vi "adad.vi"(7 "error in":errorcluster) -> (27 "error out":errorcluster)   [LabVIEW 2021]
uses:
  <vilib>/vision/NI_Vision_Development_Module.lvlib
panel:
  out "Image Out":T1(plugin-control)
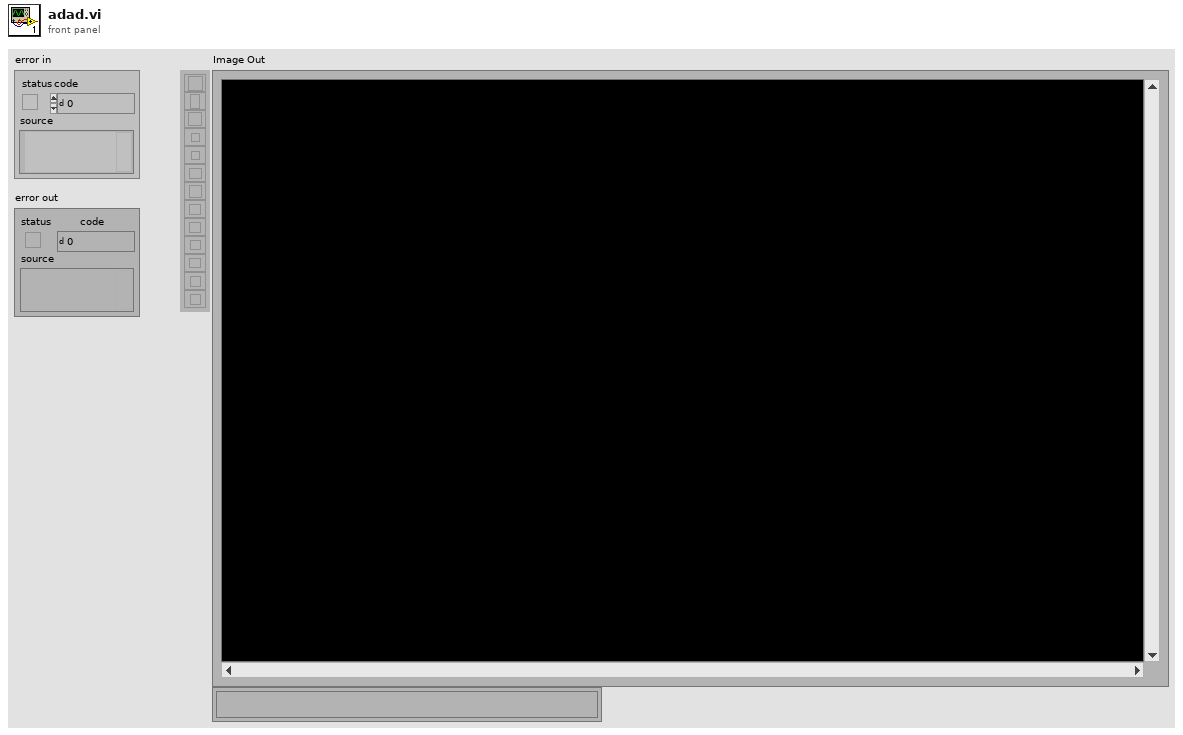
[diagram p1: front panel]
types:
  T1 = typedef "IMAQ Image.ctl" = refnum<image>
  T2 = typedef "Image Type" = u32
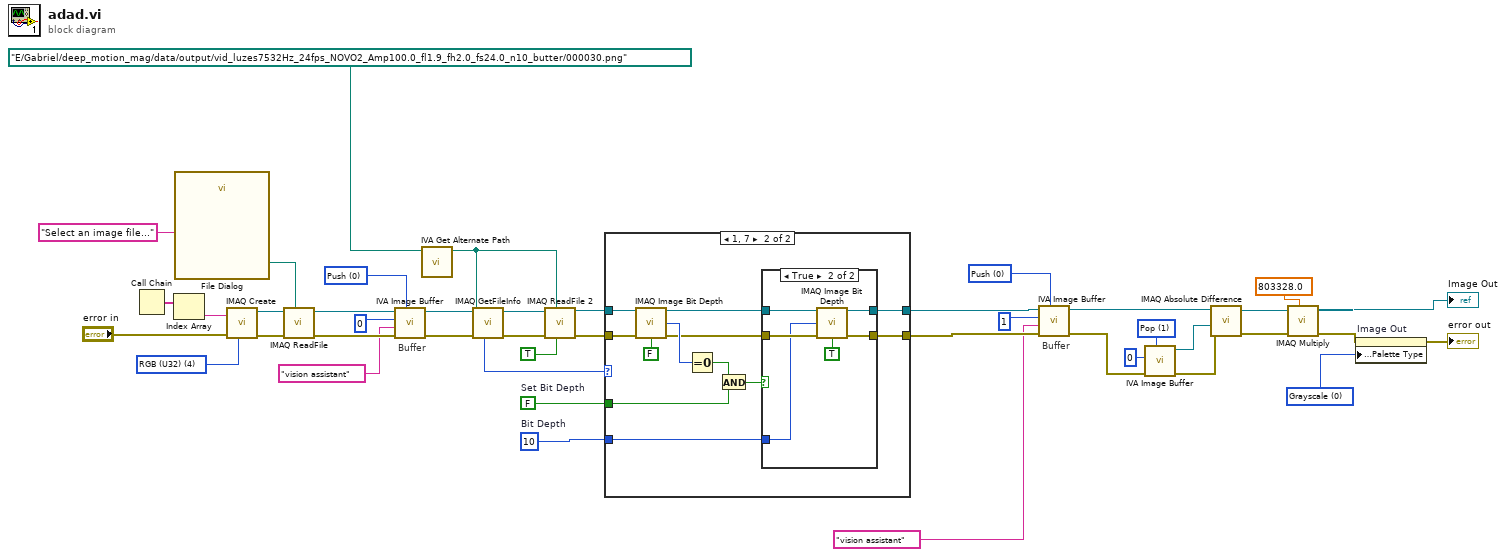
[diagram p0: block diagram]
diagram:
  w1 = u32 0 items=["Grayscale", "Binary", "Gradient", "Rainbow", "Temperature", "User Defined", "Binary 16 Bit", "Gradient 16 Bit", "Rainbow 16 Bit", "Temperature 16 Bit", "User Defined 16 Bit"] ("Palette Type")
  w12 = u16 1 items=["Push", "Pop", "Reset"] ("Function")
  w15 = u16 0 items=["Push", "Pop", "Reset"] ("Function")
  w25 = 10  # Bit Depth
  w26 = FALSE  # Set Bit Depth
  w31 = u16 0 items=["Push", "Pop", "Reset"] ("Function")
  w34 = T2 4 items=["Grayscale (U8)", "Grayscale (I16)", "Grayscale (SGL)", "Complex (CSG)", "RGB (U32)", "HSL (U32)", "RGB (U64)", "Grayscale (U16)"] ("Image Type")
  # "Buffer"
  # "Buffer"
  n1 = Call Chain() -> (call chain=w38:string[])
  n2 = Index Array(array=w38) -> (element=w37:string)  [unwired: 1 in]
  n3 = call "File Dialog"("prompt"="Select an image file...") -> ("selected path"=w35:path)  [unwired: 6 in, 8 out]
  n4 = call "IMAQ Create"("Image Name"=w37, "Image Type"=w34, "error in (no error)"="error in") -> ("New Image"=w41:T1, "error out"=w40:errorcluster)  [unwired: 1 in, 1 out]
  n5 = call "IMAQ ReadFile"("File Path"=w35, "error in (no error)"=w40, "Image"=w41) -> ("error out"=w42:errorcluster, "Image Out"=w33:T1)  [unwired: 2 in, 5 out]
  n6 = call <vilib>:"IVA Image Buffer.vi"("Function"=w31, "error in (no error)"=w42, "Prefix"="vision assistant", "Buffer #"=0, "Image In"=w33) -> ("error out"=w32:errorcluster, "Image Out"=w23:T1)  [unwired: 5 out]
  n7 = call <vilib>:"IVA Get Alternate Path.vi"("Path In"=path "E:/Gabriel/deep_motion_mag/data/output/vid_luzes7532Hz_24fps_NOVO2_Amp100.0_fl1.9_fh2.0_fs24.0_n10_butter/000030.png" ("File Path")) -> ("Path Out"=w21:path)  [unwired: 10 out]
  n8 = call "IMAQ GetFileInfo"("error in (no error)"=w32, "File Path"=w21) -> ("error out"=w19:errorcluster, "Image Type"=w27:T2)  [unwired: 8 out]
  n9 = call "IMAQ ReadFile 2"("Use File Path Image Type"=TRUE, "File Path"=w21, "error in (no error)"=w19, "Image"=w23) -> ("error out"=w20:errorcluster, "Image Out"=w22:T1)  [unwired: 3 in, 3 out]
  n10 = case shown="1, 7" w27 {
    tunnel: w22 -> [w44 w53]
    tunnel: w20 -> [w43 w52]
    tunnel: w26 -> [_ w46]
    tunnel: w25 -> [_ w56]
    tunnel: [w44 w55] -> w17
    tunnel: [w43 w54] -> w24
    frame 0, Default {
    }
    frame 1, 7 {
      n11 = call "IMAQ Image Bit Depth"("Image"=w53, "error in (no error)"=w52, "Get/Set Bit Depth? (Set)"=FALSE) -> ("Image Out"=w50:T1, "Bit Depth"=w49:u32, "error out"=w48:errorcluster)  [unwired: 10 in]
      n12 = Equal To 0?(x=w49) -> (x = 0?=w47:bool)
      n13 = And(x=w47, y=w46) -> (x .and. y?=w45:bool)
      n14 = case shown="True" w45 {
        tunnel: w50 -> [w58 w64]
        tunnel: w48 -> [w57 w63]
        tunnel: w56 -> [_ w62]
        tunnel: [w58 w61] -> w55
        tunnel: [w57 w60] -> w54
        frame False {
        }
        frame True {
          n15 = call "IMAQ Image Bit Depth"("Image"=w64, "Bit Depth (0)"=w62, "error in (no error)"=w63, "Get/Set Bit Depth? (Set)"=TRUE) -> ("Image Out"=w61:T1, "error out"=w60:errorcluster)  [unwired: 9 in, 1 out]
        }
      }
    }
  }
  n16 = call <vilib>:"IVA Image Buffer.vi"("Function"=w15, "error in (no error)"=w24, "Prefix"="vision assistant", "Buffer #"=1, "Image In"=w17) -> ("error out"=w16:errorcluster, "Image Out"=w7:T1)  [unwired: 5 out]
  n17 = call <vilib>:"IVA Image Buffer.vi"("Function"=w12, "error in (no error)"=w16, "Buffer #"=0) -> ("error out"=w9:errorcluster, "Image Out"=w10:T1)  [unwired: 2 in, 5 out]
  n18 = call "IMAQ Absolute Difference"("Image Src A"=w7, "Image Src B"=w10, "error in (no error)"=w9) -> ("Image Dst Out"=w5:T1, "error out"=w8:errorcluster)  [unwired: 2 in, 2 out]
  n19 = call "IMAQ Multiply"("Image Src A"=w5, "Constant"=sgl 803328.0, "error in (no error)"=w8) -> ("Image Dst Out"=→"Image Out":T1, "error out"=w4:errorcluster)  [unwired: 2 in, 2 out]
  n20 = property on="Image Out" class="ImageControl"(error in=w4, "Palette:Palette Type"=w1) -> (error out=→"error out":errorcluster)  [unwired: 1 in, 1 out]
